vi "lockin-monitor.vi"() -> ()   [LabVIEW 2019]
panel:
  out "waiting for lock?":bool
  in  "dt (seconds)":dbl=0.25 min=0.01 format="%#_13g"
  in  "history (seconds)":dbl=60.0 min=1.0
  out "XY Graph":cluster{dbl[], dbl[]}[](graph)
  in  "stop":bool
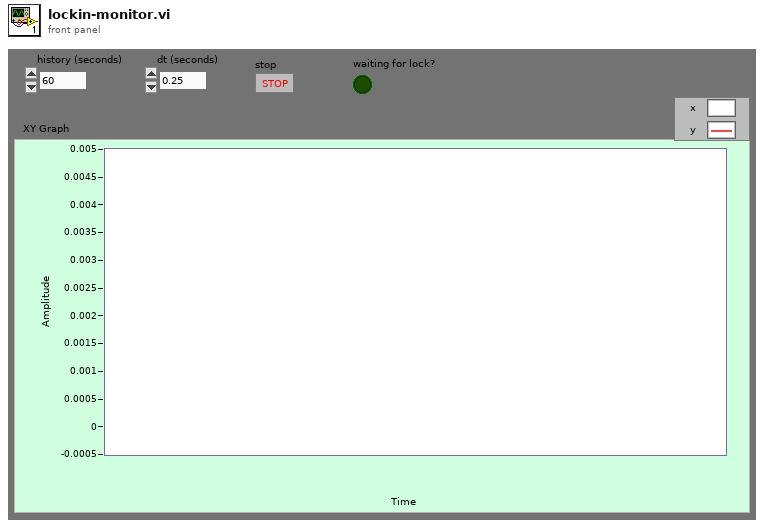
[diagram p1: front panel]
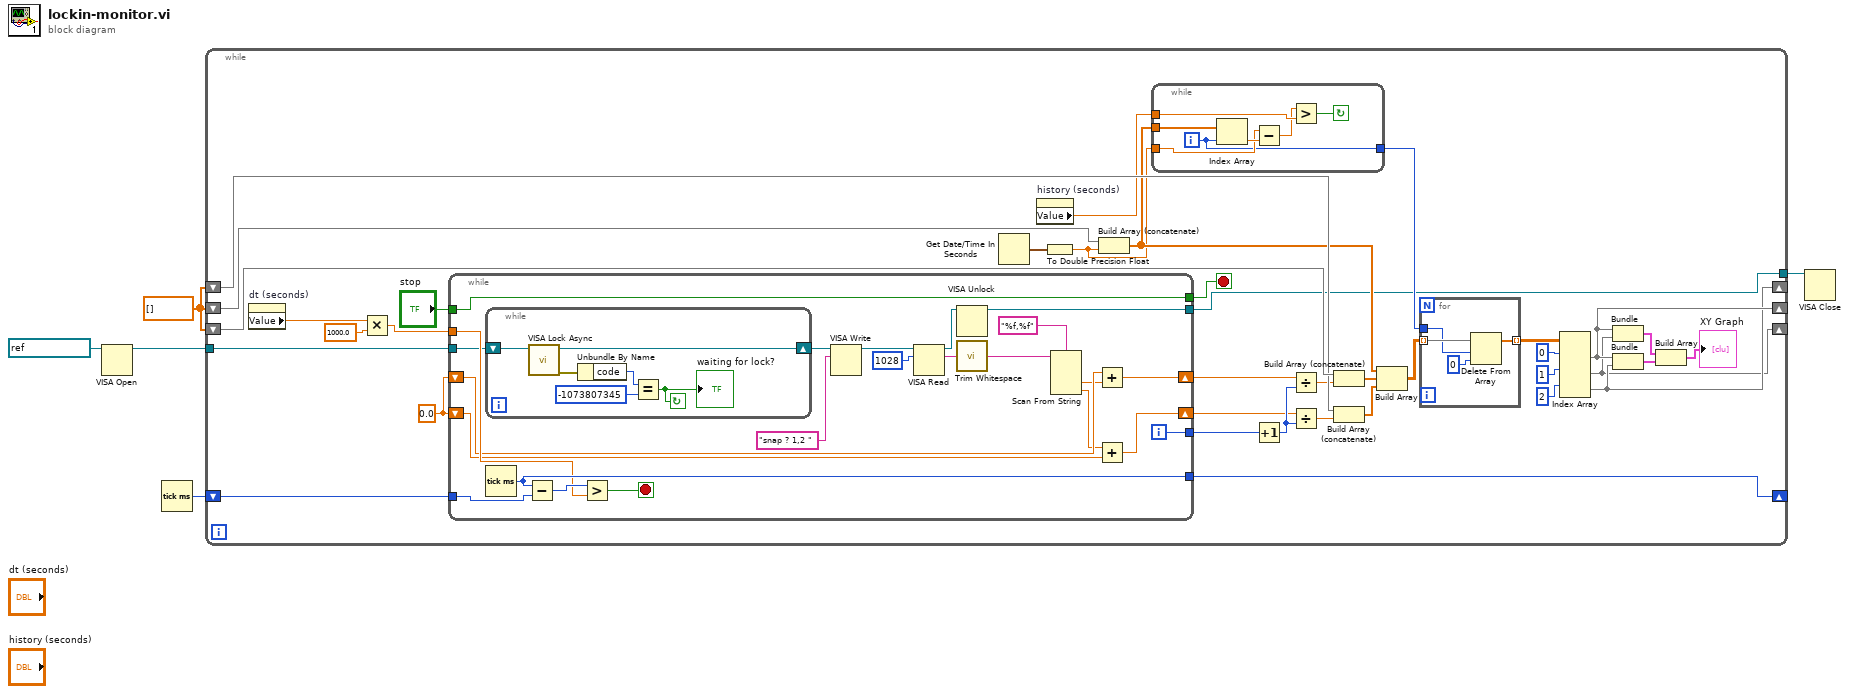
[diagram p0: block diagram]
diagram:
  w2 = dbl[] []
  n1 = VISA Open(VISA resource name=refnum<visa-resource-name> "bilt-lockin") -> (VISA resource name=w4:refnum<visa-resource-name>)  [unwired: 4 in, 1 out]
  n2 = Tick Count (ms)() -> (millisecond timer value=w1:u32)
  n3 = while {
    tunnel: w4 -> [w14]
    tunnel: [w13] -> w3
    shift-right: [w27] -> _
    shift-left: w2 -> [w41]
    shift-right: [w28] -> _
    shift-left: w2 -> [w40]
    shift-right: [w29] -> _
    shift-left: w2 -> [w39]
    shift-right: [w18] -> _
    shift-left: w1 -> [w21]
    stop <- w20 stop-if-true
    w12 = 0.0
    n4 = property on="dt (seconds)" class="DigNum (strict)"() -> ("Value"=w16:dbl)  [unwired: 2 in, 2 out]
    n5 = Multiply(x=w16, y=1000.0) -> (x*y=w15:dbl)
    n6 = while {
      tunnel: w21 -> [w65]
      tunnel: [w62] -> w20
      tunnel: "stop" -> [w62]
      tunnel: [w61] -> w18
      tunnel: w15 -> [w60]
      tunnel: w14 -> [w44]
      tunnel: [w45] -> w13
      shift-right: [w50] -> w9
      shift-left: w12 -> [w54]
      shift-right: [w49] -> w8
      shift-left: w12 -> [w51]
      tunnel: [w48] -> w11
      i -> [w48]
      stop <- w63 stop-if-true
      n7 = while {
        shift-right: [w70] -> w43
        shift-left: w44 -> [w71]
        stop <- w66 continue-if-true
        n8 = call <vilib>:"VISA Lock Async.vi"("VISA resource name"=w71) -> ("error out"=w67:errorcluster, "VISA resource name out"=w70:refnum<visa-resource-name>)  [unwired: 8 in, 1 out]
        n9 = Unbundle By Name(w67) -> ("code"=w69:i32)
        n10 = Equal?(x=w69, y=-1073807345) -> (x = y?=w66:bool)
        "waiting for lock?" <- w66
      }
      n11 = Tick Count (ms)() -> (millisecond timer value=w61:u32)
      n12 = Subtract(x=w61, y=w65) -> (x-y=w64:u32)
      n13 = Greater?(x=w64, y=w60) -> (0:w63:bool)
      n14 = VISA Write(VISA resource name=w43, write buffer="snap ? 1,2 ") -> (VISA resource name out=w59:refnum<visa-resource-name>)  [unwired: 1 in, 2 out]
      n15 = VISA Read(VISA resource name=w59, byte count=u32 1028) -> (VISA resource name out=w46:refnum<visa-resource-name>, read buffer=w58:string)  [unwired: 1 in, 2 out]
      n16 = VISA Unlock(11:w46) -> (3:w45:refnum<visa-resource-name>)  [unwired: 1 in, 1 out]
      n17 = call <vilib>:"Trim Whitespace.vi"("string"=w58) -> ("trimmed string"=w56:string)  [unwired: 1 in]
      n18 = Scan From String(format string="%f,%f", input string=w56) -> (output 1=w53:dbl, output 2=w52:dbl)  [unwired: 4 in, 3 out]
      n19 = Add(x=w54, y=w53) -> (x+y=w50:dbl)
      n20 = Add(x=w52, y=w51) -> (x+y=w49:dbl)
    }
    n21 = Get Date/Time In Seconds() -> (seconds since 1Jan1904=w42:timestamp)
    n22 = property on="history (seconds)" class="DigNum (strict)"() -> ("Value"=w23:dbl)  [unwired: 2 in, 2 out]
    n23 = To Double Precision Float(number=w42) -> (double precision float=w24:dbl)
    n24 = Build Array (concatenate)(w39, w24) -> (w25:dbl[])
    n25 = while {
      tunnel: w25 -> [w82]
      tunnel: w24 -> [w80]
      tunnel: w23 -> [w79]
      tunnel: [w76] -> w22
      i -> [w76]
      stop <- w77 continue-if-true
      n26 = Index Array(array=w82, index=w76) -> (element=w81:dbl)
      n27 = Subtract(x=w80, y=w81) -> (x-y=w78:dbl)
      n28 = Greater?(x=w78, y=w79) -> (0:w77:bool)
    }
    n29 = Increment(x=w11) -> (x+1=w10:i32)
    n30 = Divide(x=w9, y=w10) -> (x/y=w7:dbl)
    n31 = Divide(x=w8, y=w10) -> (x/y=w6:dbl)
    n32 = Build Array (concatenate)(w41, w7) -> (w36:dbl[])
    n33 = Build Array (concatenate)(w40, w6) -> (w35:dbl[])
    n34 = Build Array(w25, w36, w35) -> (w34:dbl[][])
    n35 = for {
      tunnel: w34 -> [w75] mode=indexing
      tunnel: [w74] -> w33 mode=indexing
      tunnel: w22 -> [w73]
      n36 = Delete From Array(array=w75, length=w73, index=0) -> (array with subset deleted=w74:dbl[])  [unwired: 1 out]
    }
    n37 = Index Array(array=w33, index (row) #1=0 ("index (row)"), index (row) #2=1 ("index (row)"), index (row) #3=2 ("index (row)")) -> (element #1=w29:dbl[], element #2=w27:dbl[], element #3=w28:dbl[])  [unwired: 3 in]
    n38 = Bundle(w29, w27) -> (w26:cluster{dbl[], dbl[]})  [unwired: 1 in]
    n39 = Bundle(w29, w28) -> (w38:cluster{dbl[], dbl[]})  [unwired: 1 in]
    n40 = Build Array(w26, w38) -> (→"XY Graph":cluster{dbl[], dbl[]}[])
  }
  n41 = VISA Close(VISA resource name=w3) -> ()  [unwired: 1 in, 1 out]
